vi "Get Python Range.vi"(8 "error in (no error)":errorcluster, 9 "step":i32=1, 10 "stop":i32, 11 "start":i32) -> (0 "error out":errorcluster, 3 "range":i32[](array[numeric]))   [LabVIEW 2021, in "Numeric Utilities.lvlib"]
uses:
  <vilib>/Utility/error.llb/Error Cluster From Error Code.vi
  <vilib>/ErrorRing/Error Ring.xnode
  Numeric Utilities.lvlib
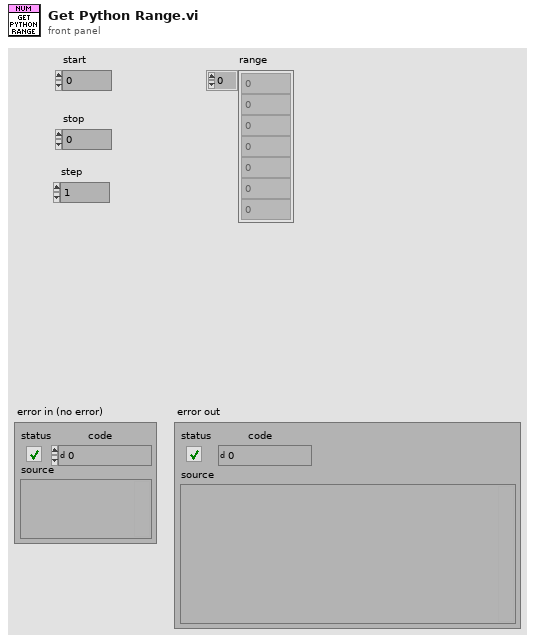
[diagram p1: front panel]
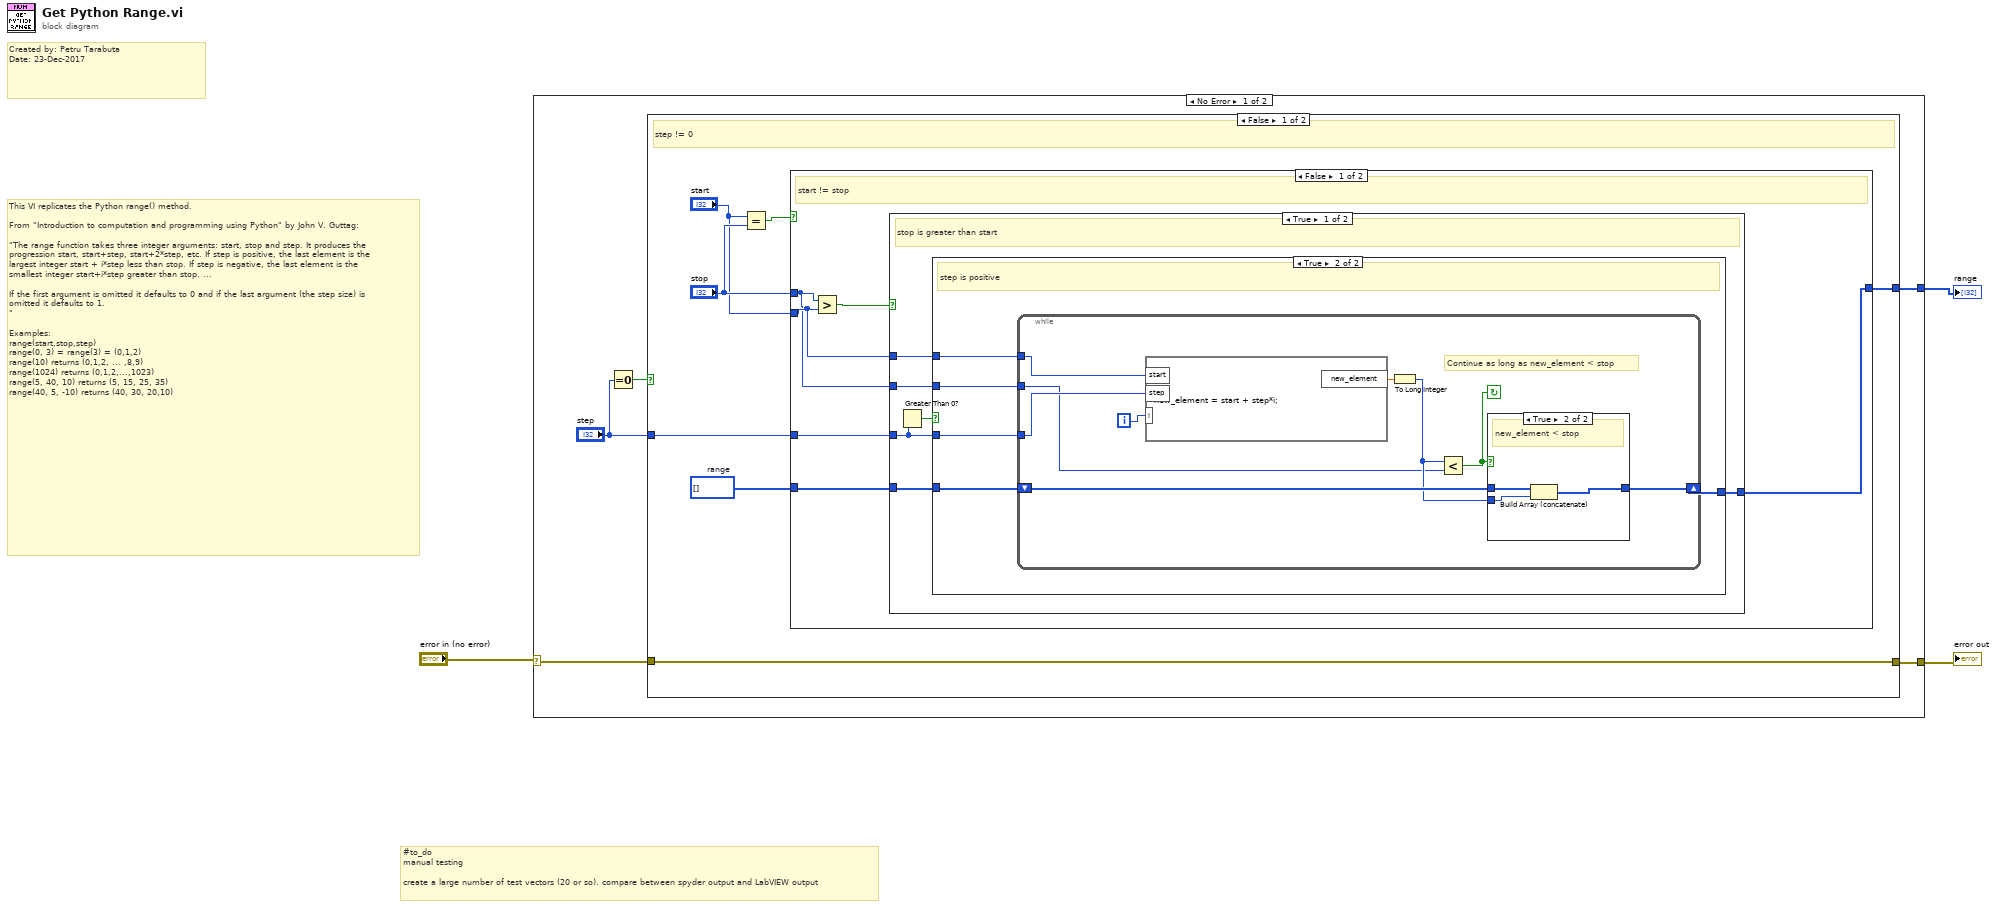
[diagram p0: block diagram]
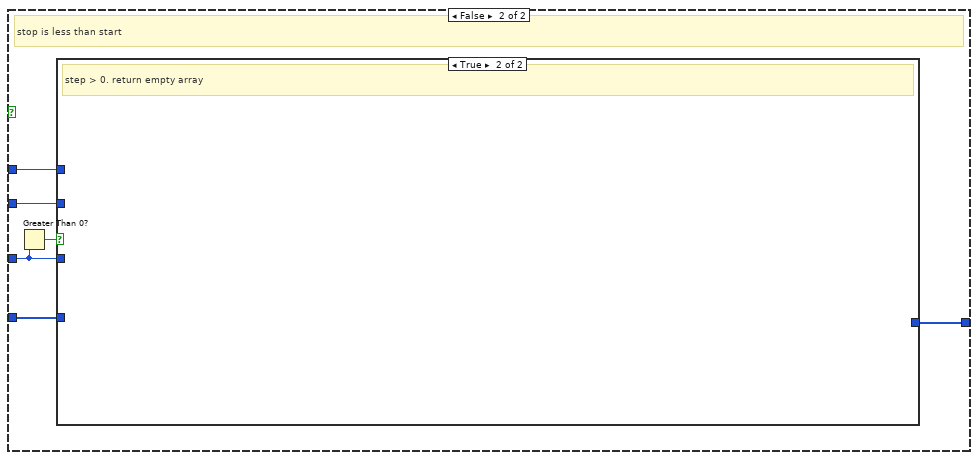
[diagram p4: hidden frame]
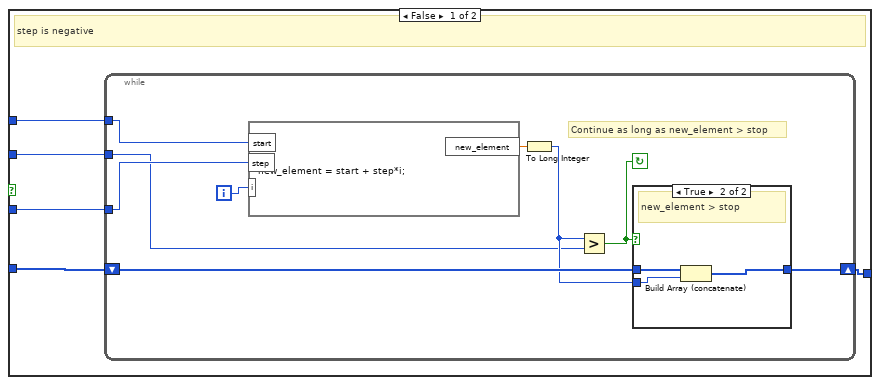
[diagram p5: hidden frame]
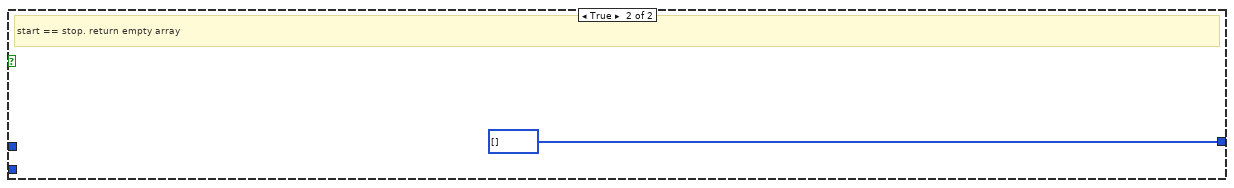
[diagram p7: hidden frame]
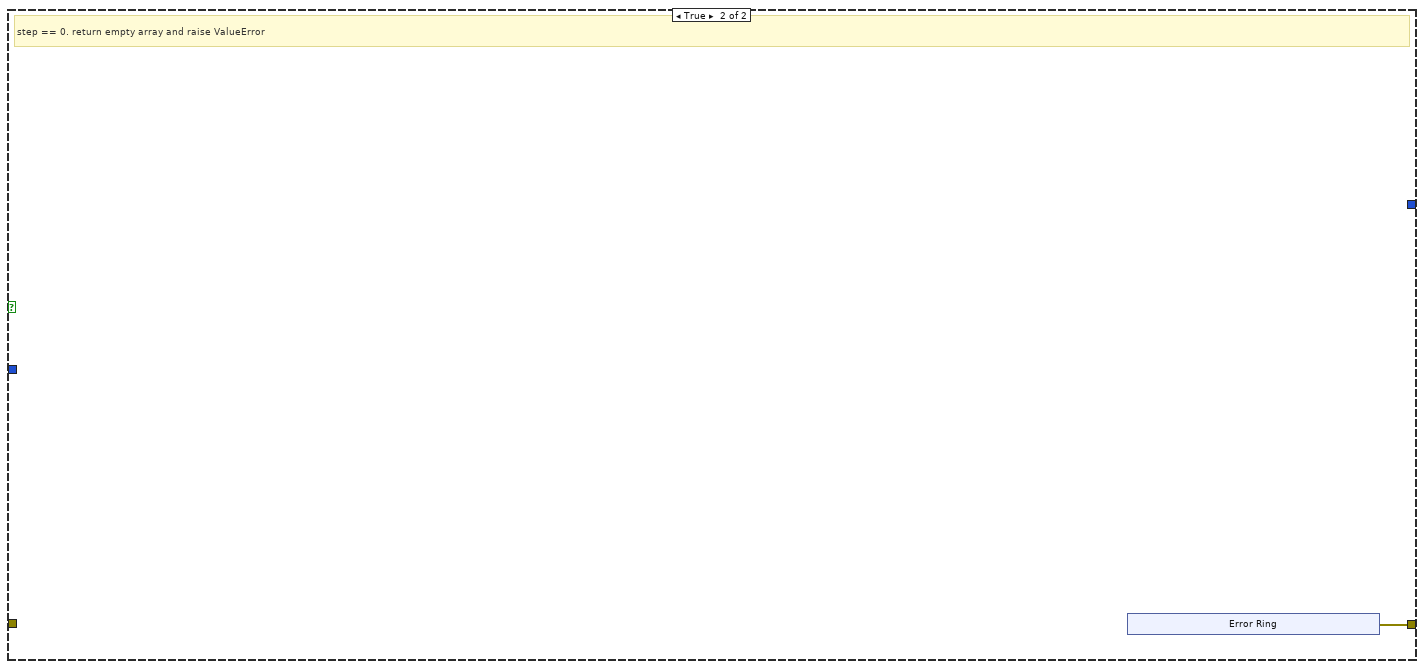
[diagram p8: hidden frame]
diagram:
  # "#to_do\nmanual testing\n\ncreate a large number of test vectors (20 or so). compare between spyder output and LabVIEW output"
  # "Created by: Petru Tarabuta\nDate: 23-Dec-2017"
  # "This VI replicates the Python range() method.\n\nFrom \"Introduction to computation and programming using Python\" by John V. Guttag:\n\n\"The range function takes three integer arguments: start, stop and step. It produces the progression start, start+step, start+2*step, etc. If step is positive, the last element is the largest integer start + i*step less than stop. If step is negative, the last element is the smallest integer start+i*step greater than stop. ... \n\nIf the first argument is omitted it defaults to 0 and if the last argument (the step size) is omitted it defaults to 1.\n\"\n\nExamples:\nrange(start,stop,step)\nrange(0, 3) = range(3) = (0,1,2)\nrange(10) returns (0,1,2, ... ,8,9)\nrange(1024) returns (0,1,2,...,1023)\nrange(5, 40, 10) returns (5, 15, 25, 35)\nrange(40, 5, -10) returns (40, 30, 20,10)"
  n1 = case shown="No Error" "error in (no error)" {
    selector: "error in (no error)" -> [w4 w77]
    tunnel: [w8 _] -> w3
    tunnel: [w5 w77] -> w1
    frame No Error {
      n2 = Equal To 0?(x="step") -> (x = 0?=w6:bool)
      n3 = case shown="False" w6 {
        tunnel: [w14 _] -> w8
        tunnel: "step" -> [w11 _]
        tunnel: [w9 w71] -> w5
        tunnel: w4 -> [w9 _]
        frame False {
          w10 = i32[] []  # range
          # "step != 0"
          n4 = Equal?(x="start", y="stop") -> (x = y?=w15:bool)
          n5 = case shown="False" w15 {
            tunnel: [w16 i32[] [] ("range")] -> w14
            tunnel: "stop" -> [w19 _]
            tunnel: "start" -> [w20 _]
            tunnel: w11 -> [w18 _]
            tunnel: w10 -> [w17 _]
            frame False {
              # "start != stop"
              n6 = Greater?(x=w19, y=w20) -> (0:w21:bool)
              n7 = case shown="True" w21 {
                tunnel: w20 -> [w27 w51]
                tunnel: w19 -> [w26 w50]
                tunnel: w18 -> [w23 w47]
                tunnel: w17 -> [w25 w49]
                tunnel: [w24 w48] -> w16
                frame True {
                  # "stop is greater than start"
                  n8 = Greater Than 0?(x=w23) -> (x > 0?=w22:bool)
                  n9 = case shown="True" w22 {
                    tunnel: w27 -> [_ w32]
                    tunnel: w26 -> [_ w31]
                    tunnel: w23 -> [_ w30]
                    tunnel: w25 -> [_ w29]
                    tunnel: [_ w28] -> w24
                    frame False {
                      # "step < 0. return empty array"
                    }
                    frame True {
                      # "step is positive"
                      n10 = while {
                        tunnel: w32 -> [w38]
                        tunnel: w31 -> [w34]
                        tunnel: w30 -> [w39]
                        shift-right: [w36] -> w28
                        shift-left: w29 -> [w41]
                        i -> [w40]
                        stop <- w33 continue-if-true
                        # "Continue as long as new_element < stop"
                        n11 = formula code="new_element = start + step*i;"("start"=w38, "step"=w39, "i"=w40) -> ("new_element"=w37:dbl)
                        n12 = To Long Integer(number=w37) -> (32bit integer=w35:i32)
                        n13 = Less?(x=w35, y=w34) -> (x < y?=w33:bool)
                        n14 = case shown="True" w33 {
                          tunnel: w41 -> [w42 w45]
                          tunnel: [w42 w44] -> w36
                          tunnel: w35 -> [_ w43]
                          frame False {
                            # "new_element > stop"
                          }
                          frame True {
                            # "new_element < stop"
                            n15 = Build Array (concatenate)(w45, w43) -> (w44:i32[])
                          }
                        }
                      }
                    }
                  }
                }
                frame False {
                  # "stop is less than start"
                  n16 = Greater Than 0?(x=w47) -> (x > 0?=w46:bool)
                  n17 = case shown="True" w46 {
                    tunnel: w51 -> [w56 _]
                    tunnel: w50 -> [w55 _]
                    tunnel: w47 -> [w54 _]
                    tunnel: w49 -> [w53 _]
                    tunnel: [w52 _] -> w48
                    frame False {
                      # "step is negative"
                      n18 = while {
                        tunnel: w56 -> [w62]
                        tunnel: w55 -> [w58]
                        tunnel: w54 -> [w63]
                        shift-right: [w60] -> w52
                        shift-left: w53 -> [w65]
                        i -> [w64]
                        stop <- w57 continue-if-true
                        # "Continue as long as new_element > stop"
                        n19 = formula code="new_element = start + step*i;"("start"=w62, "step"=w63, "i"=w64) -> ("new_element"=w61:dbl)
                        n20 = To Long Integer(number=w61) -> (32bit integer=w59:i32)
                        n21 = Greater?(x=w59, y=w58) -> (0:w57:bool)
                        n22 = case shown="True" w57 {
                          tunnel: w65 -> [w66 w69]
                          tunnel: [w66 w68] -> w60
                          tunnel: w59 -> [_ w67]
                          frame False {
                            # "new_element < stop"
                          }
                          frame True {
                            # "new_element > stop"
                            n23 = Build Array (concatenate)(w69, w67) -> (w68:i32[])
                          }
                        }
                      }
                    }
                    frame True {
                      # "step > 0. return empty array"
                    }
                  }
                }
              }
            }
            frame True {
              # "start == stop. return empty array"
            }
          }
        }
        frame True {
          # "step == 0. return empty array and raise ValueError"
          n24 = xnode "Error Ring"() -> ("error out"=w71:errorcluster)
        }
      }
    }
    frame Error {
    }
  }
  "error out" <- w1
  "range" <- w3
